vi "ProcessHandshakeRequest.vi"(0 "HTTP Headers":string, 11 "error in (no error)":errorcluster) -> (3 "Host":string, 4 "Is Websocket Request?":bool, 6 "URI":string, 8 "Resource Name":string, 10 "Sec-WebSocket-Key":string, 14 "Headers Out":variant, 15 "error out":errorcluster)   [LabVIEW 2016, in "LV WebSockets.lvlib"]
doc: "Converts the raw HTTP header string into it's main component parts needed to check if the incoming connection is a WS connection. The additional headers are returned in a variant lookup table.\nWebSockets 1.6.0.22\nSam Sharp - MediaMongrels Ltd\nCopyright (c) 2016, MediaMongrels Ltd"
uses:
  LV WebSockets.lvlib
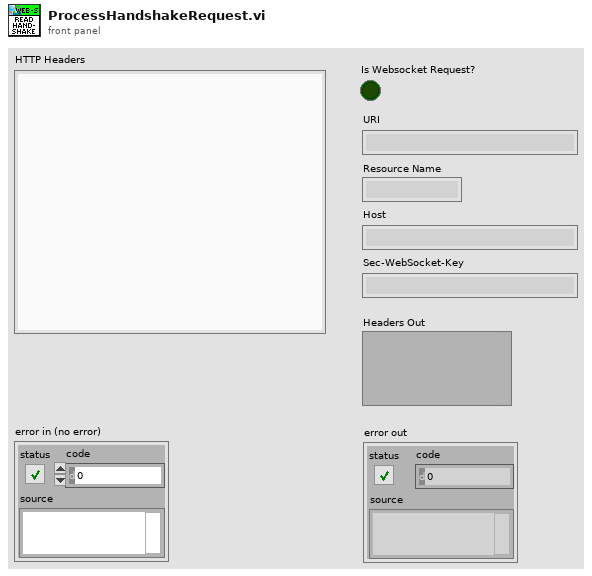
[diagram p1: front panel]
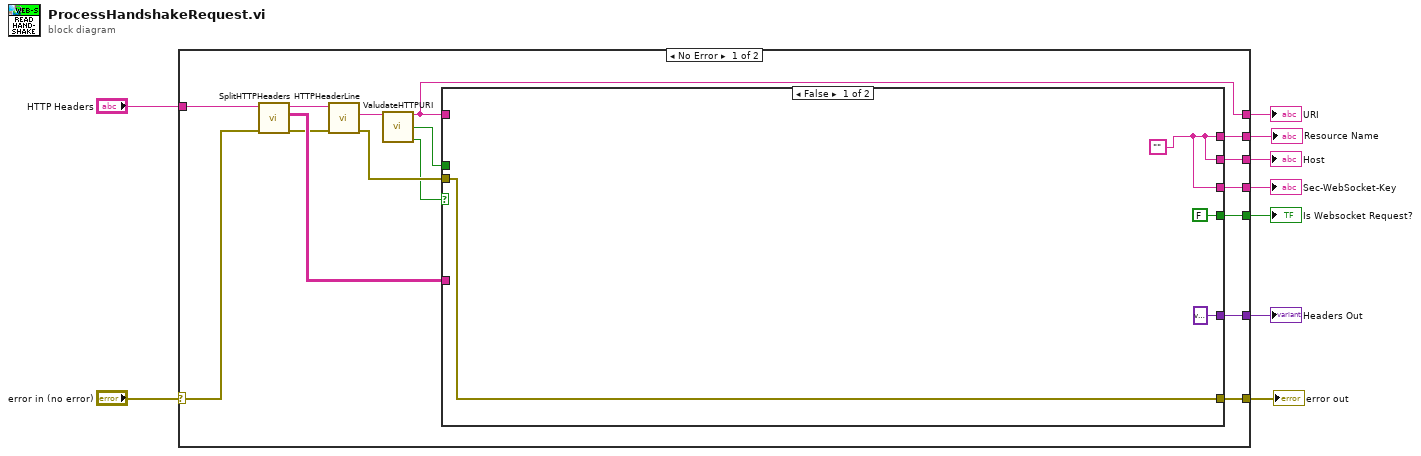
[diagram p0: block diagram]
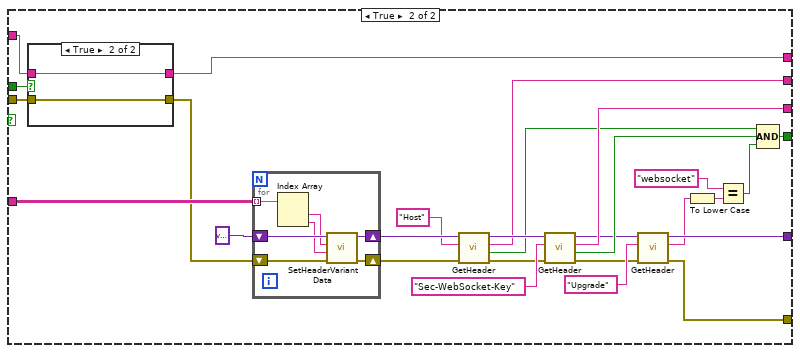
[diagram p2: hidden frame]
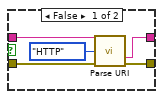
[diagram p3: hidden frame]
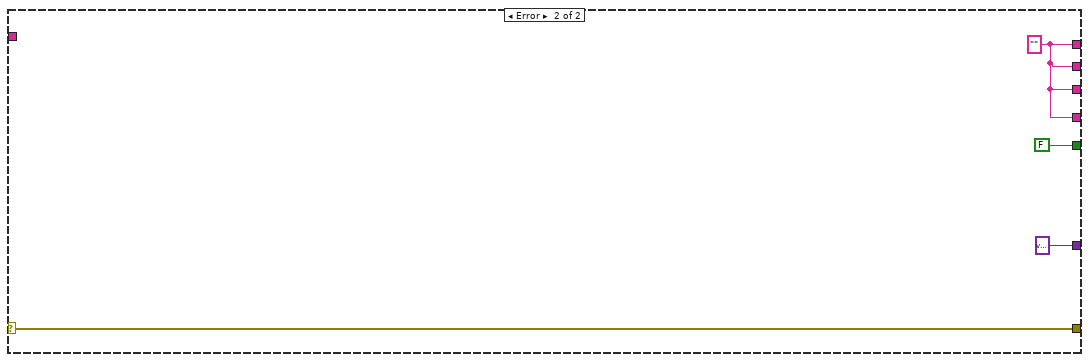
[diagram p4: hidden frame]
diagram:
  n1 = case shown="No Error" "error in (no error)" {
    selector: "error in (no error)" -> [w18 w74]
    tunnel: "HTTP Headers" -> [w25 _]
    tunnel: [w12 w71] -> w8
    tunnel: [w22 w71] -> w7
    tunnel: [w21 w71] -> w6
    tunnel: [w20 variant ("Headers Out")] -> w5
    tunnel: [w19 FALSE] -> w4
    tunnel: [w16 w74] -> w2
    tunnel: [w15 w71] -> w1
    frame No Error {
      n2 = call "SplitHTTPHeaders.vi"("error in (no error)"=w18, "HTTP Header String"=w25) -> ("error out"=w17:errorcluster, "Headers Array"=w23:string[][], "HTTP Request"=w24:string)  [unwired: 7 in]
      n3 = call "HTTPHeaderLine.vi"("error in (no error)"=w17, "HTTP Request Line"=w24) -> ("error out"=w14:errorcluster, "Request URI"=w13:string)  [unwired: 6 in, 2 out]
      n4 = call "ValudateHTTPURI.vi"("HTTP URI"=w13) -> ("HTTP URI Out"=w12:string, "Relative"=w11:bool, "Valid HTTP URI"=w10:bool)  [unwired: 12 in]
      n5 = case shown="False" w10 {
        tunnel: w23 -> [_ w56]
        tunnel: [w29 w51] -> w22
        tunnel: [w29 w49] -> w21
        tunnel: [variant ("Headers Out") w45] -> w20
        tunnel: [FALSE w41] -> w19
        tunnel: [w26 w38] -> w16
        tunnel: [w29 w34] -> w15
        tunnel: w14 -> [w26 w33]
        tunnel: w12 -> [_ w31]
        tunnel: w11 -> [_ w30]
        frame False {
          w29 = ""
        }
        frame True {
          n6 = case shown="True" w30 {
            tunnel: w31 -> [w61 w63]
            tunnel: [w59 w63] -> w34
            tunnel: w33 -> [w60 w62]
            tunnel: [w58 w62] -> w32
            frame False {
              n7 = call "Parse URI.vi"("URI"=w61, "URI type (WS)"=enum16{"WS", "HTTP"}."HTTP", "error in"=w60) -> ("Resource Name"=w59:string, "error out"=w58:errorcluster)  [unwired: 6 in, 5 out]
            }
            frame True {
            }
          }
          n8 = for {
            tunnel: w56 -> [w70] mode=indexing
            shift-right: [w69] -> w54
            shift-left: variant -> [w66]
            shift-right: [w68] -> w37
            shift-left: w32 -> [w67]
            n9 = Index Array(array=w70) -> (element #1=w65:string, element #2=w64:string)  [unwired: 2 in]
            n10 = call "SetHeaderVariantData.vi"("error in (no error)"=w67, "Value"=w64, "Name"=w65, "Variant in"=w66) -> ("error out"=w68:errorcluster, "Variant out"=w69:variant)  [unwired: 6 in]
          }
          n11 = call "GetHeader.vi"("error in (no error)"=w37, "Name"="Host" ("name"), "Headers In"=w54) -> ("error out"=w40:errorcluster, "Found?"=w48:bool, "Data"=w51:string, "Headers Out"=w52:variant)  [unwired: 5 in]
          n12 = call "GetHeader.vi"("error in (no error)"=w40, "Name"="Sec-WebSocket-Key", "Headers In"=w52) -> ("error out"=w39:errorcluster, "Found?"=w47:bool, "Data"=w49:string, "Headers Out"=w46:variant)  [unwired: 5 in]
          n13 = call "GetHeader.vi"("error in (no error)"=w39, "Name"="Upgrade", "Headers In"=w46) -> ("error out"=w38:errorcluster, "Data"=w36:string, "Headers Out"=w45:variant)  [unwired: 5 in, 1 out]
          n14 = To Lower Case(string=w36) -> (all lower case string=w35:string)
          n15 = Equal?(x="websocket", y=w35) -> (x = y?=w42:bool)
          n16 = Compound Arithmetic op=AND(w48, w47, w42) -> (w41:bool)
        }
      }
    }
    frame Error {
      w71 = "" ("Request URI")
    }
  }
  "Host" <- w7
  "URI" <- w8
  "Sec-WebSocket-Key" <- w6
  "Is Websocket Request?" <- w4
  "Headers Out" <- w5
  "error out" <- w2
  "Resource Name" <- w1
